vi "test_TCP Clear Error.vi"(8 "error in (no error)":errorcluster, 11 "TestCase in":refnum<class "Ethernet Protocol Tests.lvclass">) -> (0 "error out":errorcluster, 3 "TestCase out":refnum<class "Ethernet Protocol Tests.lvclass">)   [LabVIEW 2019, in "Ethernet Protocol Tests.lvclass"]
uses:
  Ethernet Protocol Tests.lvclass
  TCP/TCP.lvclass
  TCP/TCP.lvclass/TCP.ctl
  <vilib>/addons/_JKI Toolkits/VI Tester/TestCase.llb/TestCase.lvclass
  C:/Program Files (x86)/National Instruments/LabVIEW 2019/vi.lib/addons/_JKI Toolkits/VI Tester/TestCase.llb/TestCase.lvclass
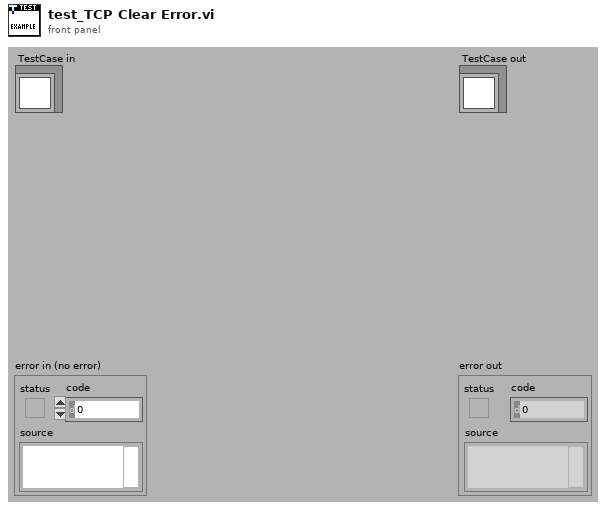
[diagram p1: front panel]
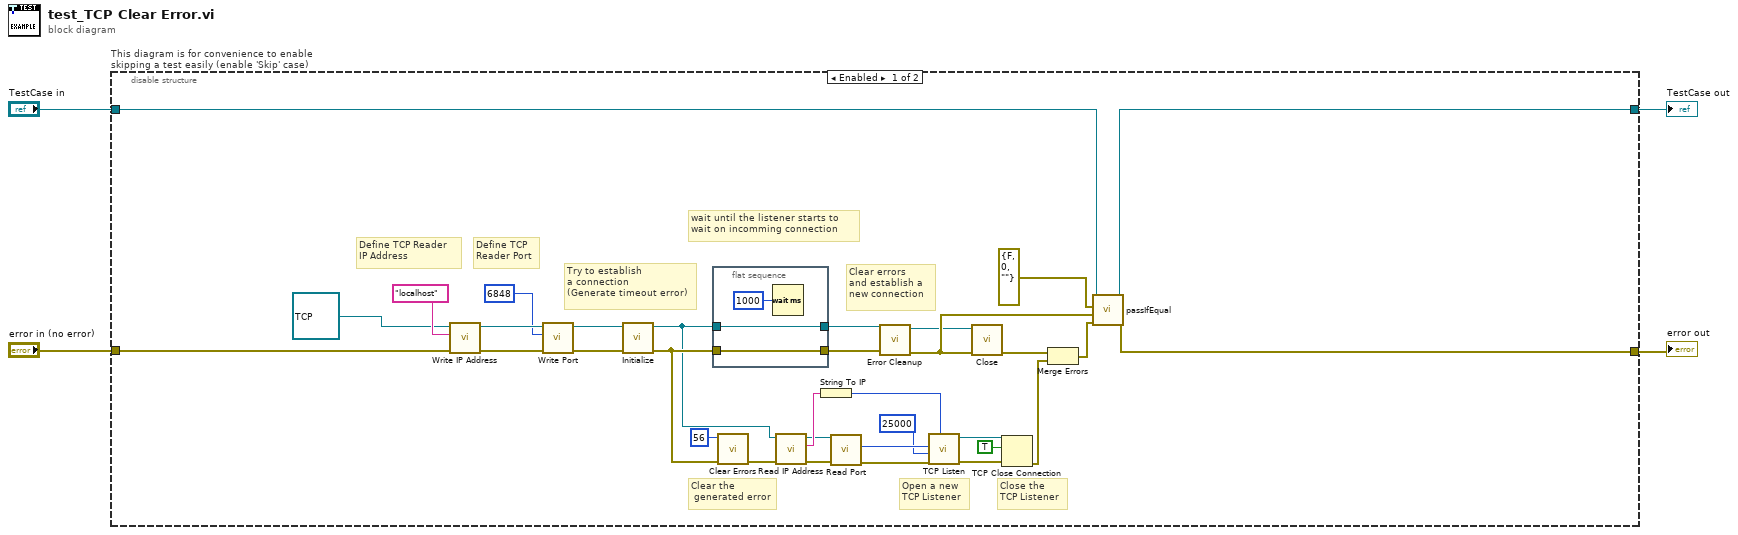
[diagram p0: block diagram]
diagram:
  n1 = disable-structure "This diagram is for convenience to enable skipping a test easily (enable 'Skip' case)" shown="Enabled" {
    disable-tunnel: "TestCase in" -> [w37 w44]
    disable-tunnel: [w9 w42] -> w1
    disable-tunnel: [w8 w43] -> w3
    disable-tunnel: "error in (no error)" -> [w31 w41]
    frame Enabled {
      # "Clear the\n generated error"
      # "Close the \nTCP Listener"
      # "Open a new \nTCP Listener"
      # "Clear errors \nand establish a \nnew connection"
      # "Try to establish \na connection\n(Generate timeout error)"
      # "wait until the listener starts to\nwait on incomming connection"
      # "Define TCP \nReader Port"
      # "Define TCP Reader \nIP Address"
      n2 = call "Write IP Address.vi"("error in (no error)"=w31, "IP Address"="localhost", "Ethernet in"=refnum<class "TCP.lvclass"> refnum ("Protocols.lvlib:TCP.lvclass")) -> ("error out"=w34:errorcluster, "Ethernet out"=w35:refnum<class "TCP.lvclass">)  [unwired: 7 in]
      n3 = call "Write Port.vi"("error in (no error)"=w34, "Port"=u16 6848, "Ethernet in"=w35) -> ("error out"=w29:errorcluster, "Ethernet out"=w28:refnum<class "TCP.lvclass">)  [unwired: 7 in]
      n4 = call-dynamic "Initialize.vi"("error in (no error)"=w29, "Ethernet in"=w28) -> ("error out"=w17:errorcluster, "Ethernet out"=w16:refnum<class "TCP.lvclass">)  [unwired: 8 in]
      n5 = flat-sequence {
        tunnel: w17 -> [w40]
        tunnel: w16 -> [w39]
        tunnel: [w40] -> w20
        tunnel: [w39] -> w19
        frame #0 {
          n6 = Wait (ms)(milliseconds to wait=u32 1000) -> ()  [unwired: 1 out]
        }
      }
      n7 = call <vilib>:"Clear Errors.vi"("error in (no error)"=w17, "specific error code to clear (0: all)"=56) -> ("error out"=w18:errorcluster)  [unwired: 4 in, 1 out]
      n8 = call "Read IP Address.vi"("error in (no error)"=w18, "Ethernet in"=w16) -> ("error out"=w25:errorcluster, "IP Address"=w27:string, "Ethernet out"=w24:refnum<class "TCP.lvclass">)  [unwired: 7 in]
      n9 = String To IP(1:w27) -> (0:w26:u32)
      n10 = call "Read Port.vi"("error in (no error)"=w25, "Ethernet in"=w24) -> ("error out"=w23:errorcluster, "Port"=w22:u16)  [unwired: 7 in, 1 out]
      n11 = call-dynamic "Error Cleanup.vi"("error in (no error)"=w20, "Ethernet in"=w19) -> ("error out"=w7:errorcluster, "Ethernet out"=w6:refnum<class "TCP.lvclass">)  [unwired: 8 in]
      n12 = call <vilib>:"TCP Listen.vi"("net address"=w26, "error in (no error)"=w23, "timeout ms (wait forever: -1)"=25000, "port"=w22) -> ("error out"=w14:errorcluster, "connection ID"=w13:refnum<k5>)  [unwired: 3 in, 3 out]
      n13 = call-dynamic "Close.vi"("error in (no error)"=w7, "Ethernet in"=w6) -> ("error out"=w5:errorcluster)  [unwired: 8 in, 1 out]
      n14 = TCP Close Connection(connection ID=w13, abort (F)=TRUE, error in (no error)=w14) -> (error out=w11:errorcluster)  [unwired: 1 out]
      n15 = Merge Errors(w5, w11) -> (w10:errorcluster)
      n16 = call-dynamic "passIfEqual.vi"("error in (no error)"=w10, "y"=w7, "x"=errorcluster {"status"=FALSE, "code"=0, "source"=""} ("error constant"), "TestCase in"=w37) -> ("error out"=w8:errorcluster, "TestCase out"=w9:refnum<class "Ethernet Protocol Tests.lvclass">)  [unwired: 6 in]
    }
    frame Disabled {
      # "skip test result while test is under development"
      n17 = call <vilib>:"skip.vi"("error in (no error)"=w41, "TestCase in"=w44) -> ("error out"=w43:errorcluster, "TestCase out"=w42:refnum<class "Ethernet Protocol Tests.lvclass">)  [unwired: 8 in]
    }
  }
  "error out" <- w3
  "TestCase out" <- w1
